vi "probe.vi"(1 "Degrees out 2":i32, 2 "Degrees out":i32, 3 "output":dbl) -> (0 "Waveform Chart":T1(graph))   [LabVIEW 2009]
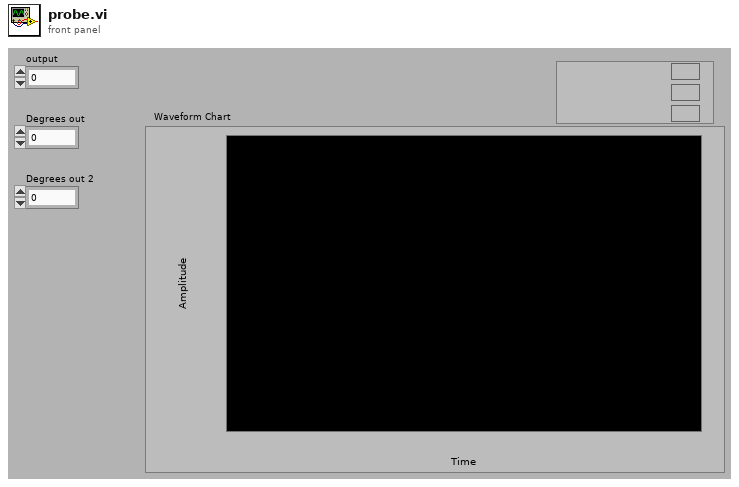
[diagram p1: front panel]
types:
  T1 = cluster{"output":dbl, "Degrees out":i32, "Degrees out":i32}
  T2 = cluster{"output":dbl, "Degrees out":i32, "Degrees out 2":i32}
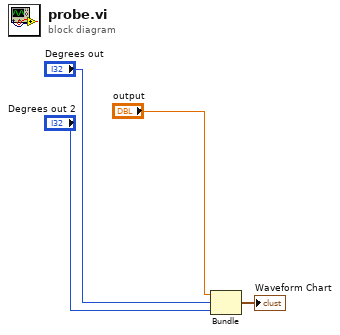
[diagram p0: block diagram]
diagram:
  n1 = Bundle("output"="output", "Degrees out"="Degrees out", "Degrees out 2"="Degrees out 2") -> (→"Waveform Chart":T2)  [unwired: 1 in]
